vi "FG Sensor Buffers SICK.vi"(2 "FG Actions (Read)":T2, 3 "SICK Buffer in":T1) -> (1 "SICK Buffer out":T1)   [LabVIEW 2009]
uses:
  Actions for FG's.ctl
  TypeDefs/Sensor TypeDefs/SICK Array.ctl
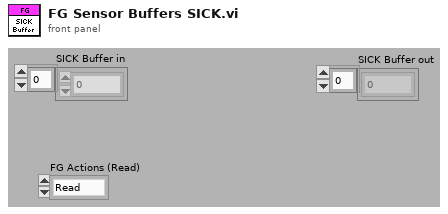
[diagram p1: front panel]
types:
  T1 = typedef "SICK Array.ctl" = u16[]
  T2 = typedef "Actions for FG's.ctl" = enum16{"Read", "Write"}
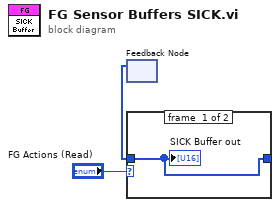
[diagram p0: block diagram]
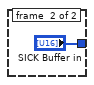
[diagram p2: hidden frame]
diagram:
  n1 = feedback #1() -> (w1:T1)  [unwired: 1 in]
  n2 = case shown="\"Read\", Default" "FG Actions (Read)" {
    tunnel: w1 -> [w4 _]
    tunnel: [w4 "SICK Buffer in"] -> w2
    frame #0 {
      "SICK Buffer out" <- w4
    }
    frame #1 {
    }
  }
